vi "Read Air Flow.vi"(7 "Flow units":enum16{"scfm", "l/s"}(ring), 8 "error in (no error)":errorcluster, 11 "VISA resource name":refnum<visa-resource-name>) -> (0 "error out":errorcluster, 2 "Air Flow":dbl format="%#.1g", 3 "VISA resource name out":refnum<visa-resource-name>, 5 "Flow units out":enum16{"scfm", "l/s"}(ring))   [LabVIEW 2010, in "Temptronic TP04300.lvlib"]
doc: "This VI reads the current air flow in scfm."
uses:
  Temptronic TP04300.lvlib
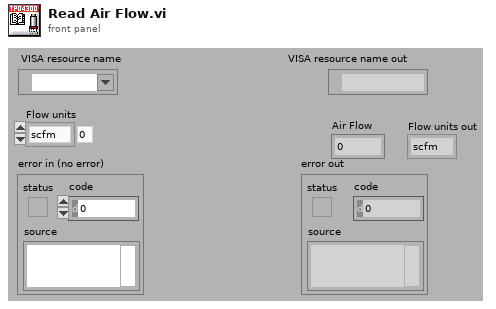
[diagram p1: front panel]
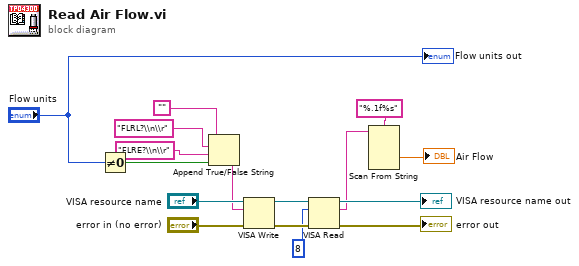
[diagram p0: block diagram]
diagram:
  n1 = Not Equal To 0?(x="Flow units") -> (x != 0?=w5:bool)
  n2 = Append True/False String(1:w5, 2:"FLRE?\\n\\r" ("multi-line string"), 3:"FLRL?\\n\\r" ("multi-line string"), 4:"") -> (0:w1:string)
  n3 = VISA Write(VISA resource name="VISA resource name", write buffer=w1, error in (no error)="error in (no error)") -> (VISA resource name out=w12:refnum<visa-resource-name>, error out=w14:errorcluster)  [unwired: 1 out]
  n4 = VISA Read(VISA resource name=w12, byte count=u32 8, error in (no error)=w14) -> (VISA resource name out=→"VISA resource name out":refnum<visa-resource-name>, read buffer=w8:string, error out=→"error out":errorcluster)  [unwired: 1 out]
  n5 = Scan From String(format string="%.1f%s" ("multi-line string"), input string=w8) -> (output 1=→"Air Flow":dbl)  [unwired: 5 in, 3 out]
  "Flow units out" <- "Flow units"
